vi "Get Command FIFO.vi"(11 "Thread in":refnum<class "Thread.lvclass">) -> (2 "command FIFO":refnum<k33>, 3 "Thread out":refnum<class "Thread.lvclass">)   [LabVIEW 2017, in "DSF Core.lvlib" / "Thread.lvclass"]
uses:
  Thread.lvclass
  Thread Command.ctl
  Thread.lvclass/Thread.ctl
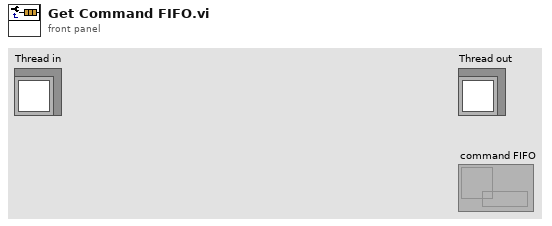
[diagram p1: front panel]
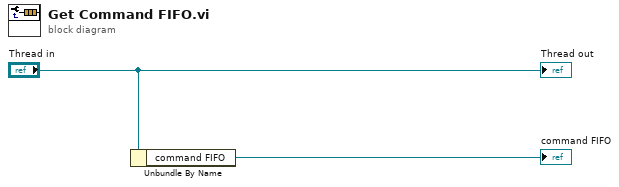
[diagram p0: block diagram]
diagram:
  n1 = Unbundle By Name("Thread in") -> ("command FIFO"=→"command FIFO":refnum<k33>)
  "Thread out" <- "Thread in"
